vi "digital_bandstop.vi"() -> ()   [LabVIEW 2023]
uses:
  <vilib>/addons/Biomedical/Biosignal Measurements/EEG/EEG FFT Spectrum (Waveform).vi
  <vilib>/addons/Biomedical/NI_BMTK_Measurements.lvlib
panel:
  out "EEG FFT Spectrum before filtering":cluster{"f0":dbl, "df":dbl, "S(f)":dbl[]}(graph)
  out "After High-pass: fc = 1 Hz":dynamicdata(graph)
  out "EEG Signal":dynamicdata(graph)
  out "Gamma Wave FFT Spectrum":cluster{"f0":dbl, "df":dbl, "S(f)":dbl[]}(graph)
  out "Beta Wave FFT Spectrum":cluster{"f0":dbl, "df":dbl, "S(f)":dbl[]}(graph)
  out "Alpha Wave FFT Spectrum":cluster{"f0":dbl, "df":dbl, "S(f)":dbl[]}(graph)
  out "Theta Wave FFT Spectrum":cluster{"f0":dbl, "df":dbl, "S(f)":dbl[]}(graph)
  out "Delta Wave FFT Spectrum":cluster{"f0":dbl, "df":dbl, "S(f)":dbl[]}(graph)
  out "FFT Spectrum":cluster{"f0":dbl, "df":dbl, "S(f)":dbl[]}(graph)
  out "Delta Wave":dynamicdata(graph)
  out "Gamma Wave":dynamicdata(graph)
  out "Beta Wave":dynamicdata(graph)
  out "Alpha Wave":dynamicdata(graph)
  out "Theta Wave":dynamicdata(graph)
  out "After Band-stop: fc = 50 Hz":dynamicdata(graph)
  out "After Low-pass: fc = 31 Hz":dynamicdata(graph)
  in  "stop":bool
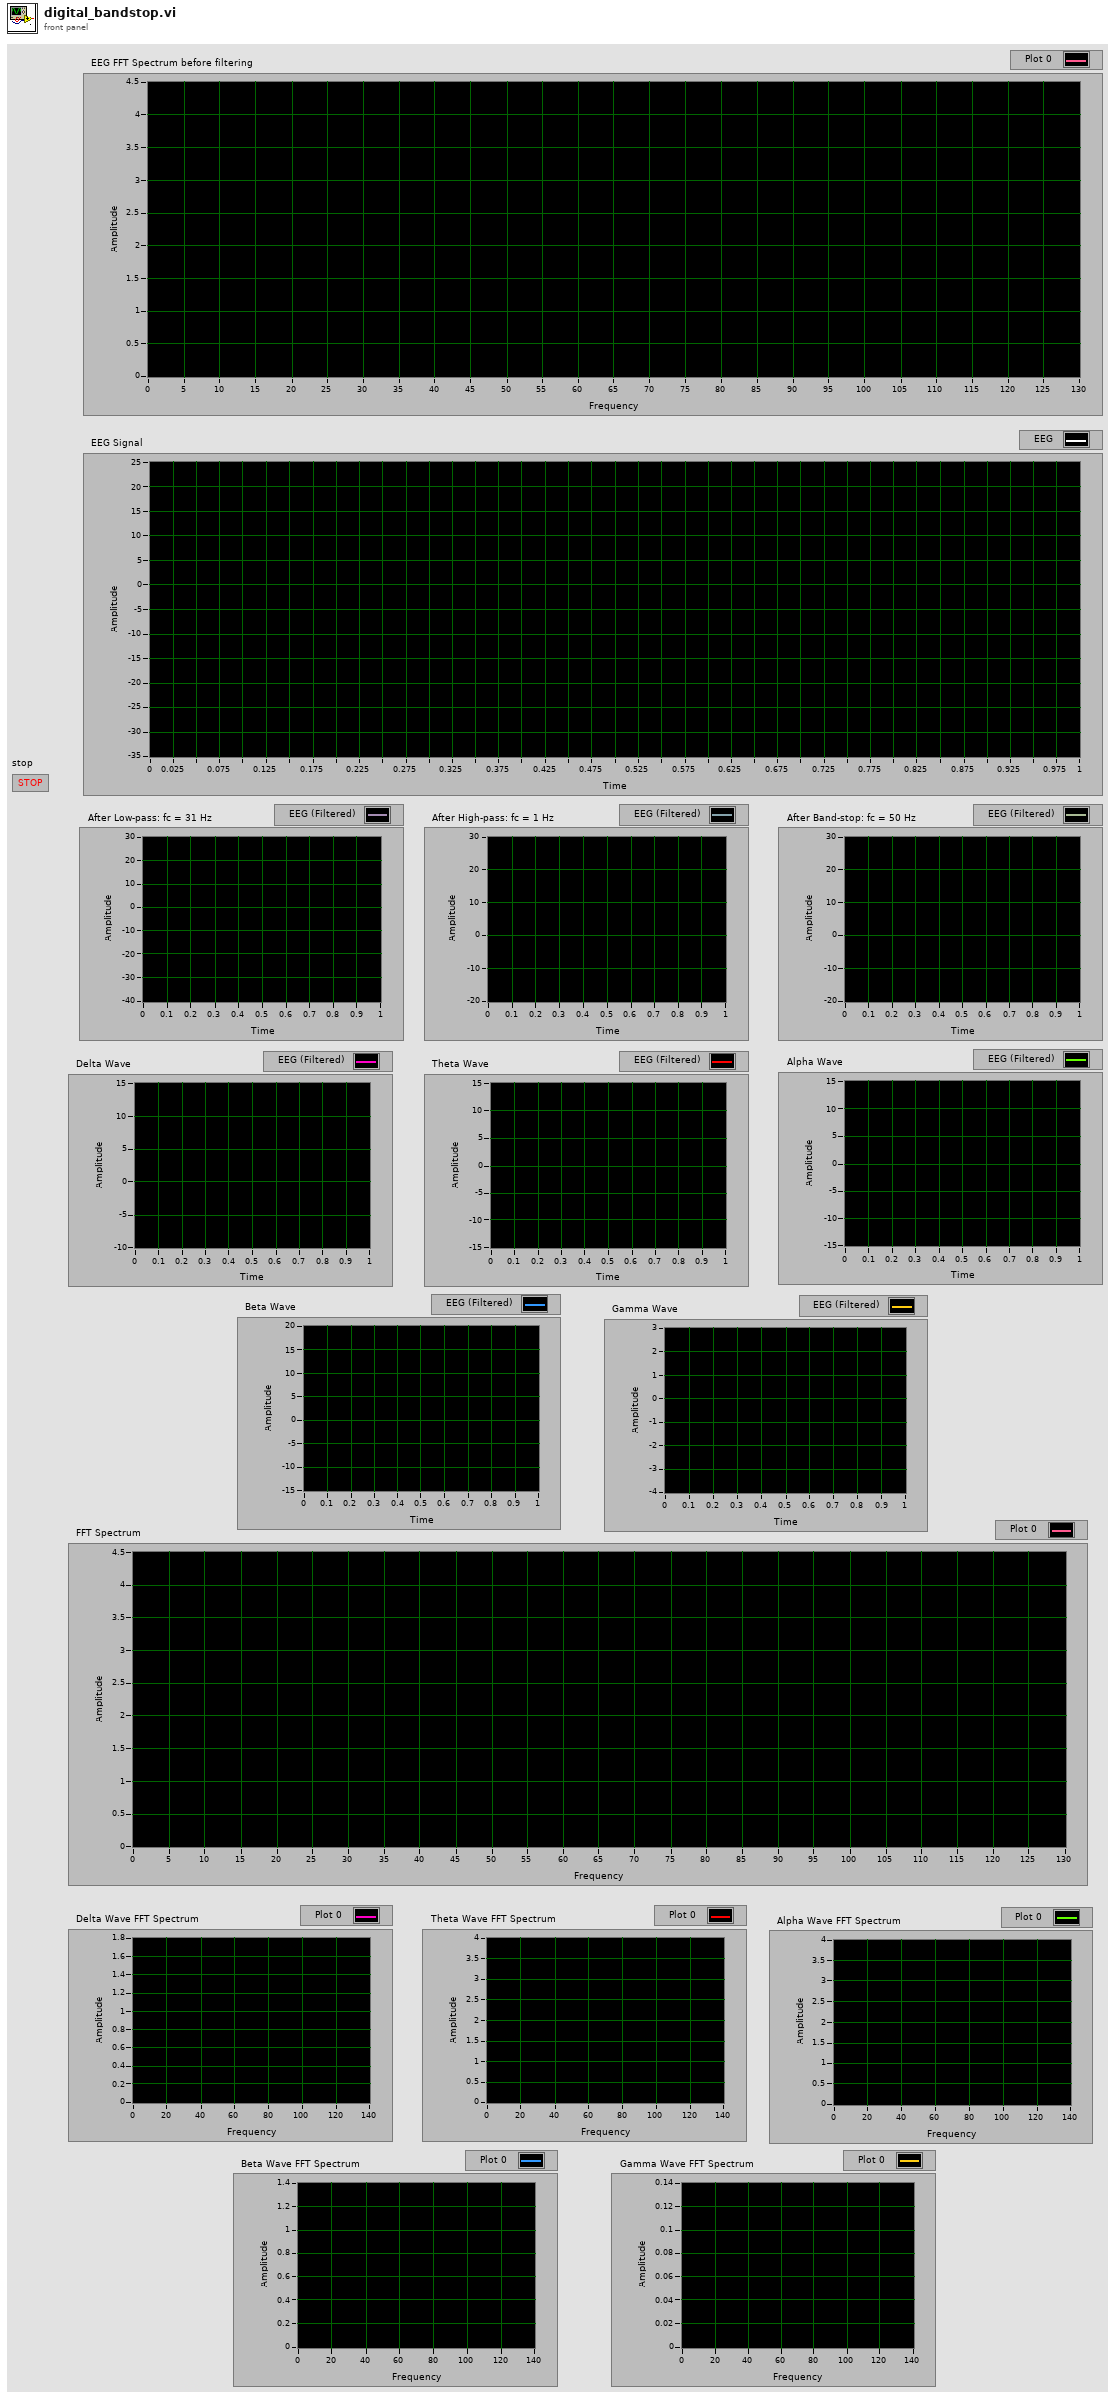
[diagram p1: front panel]
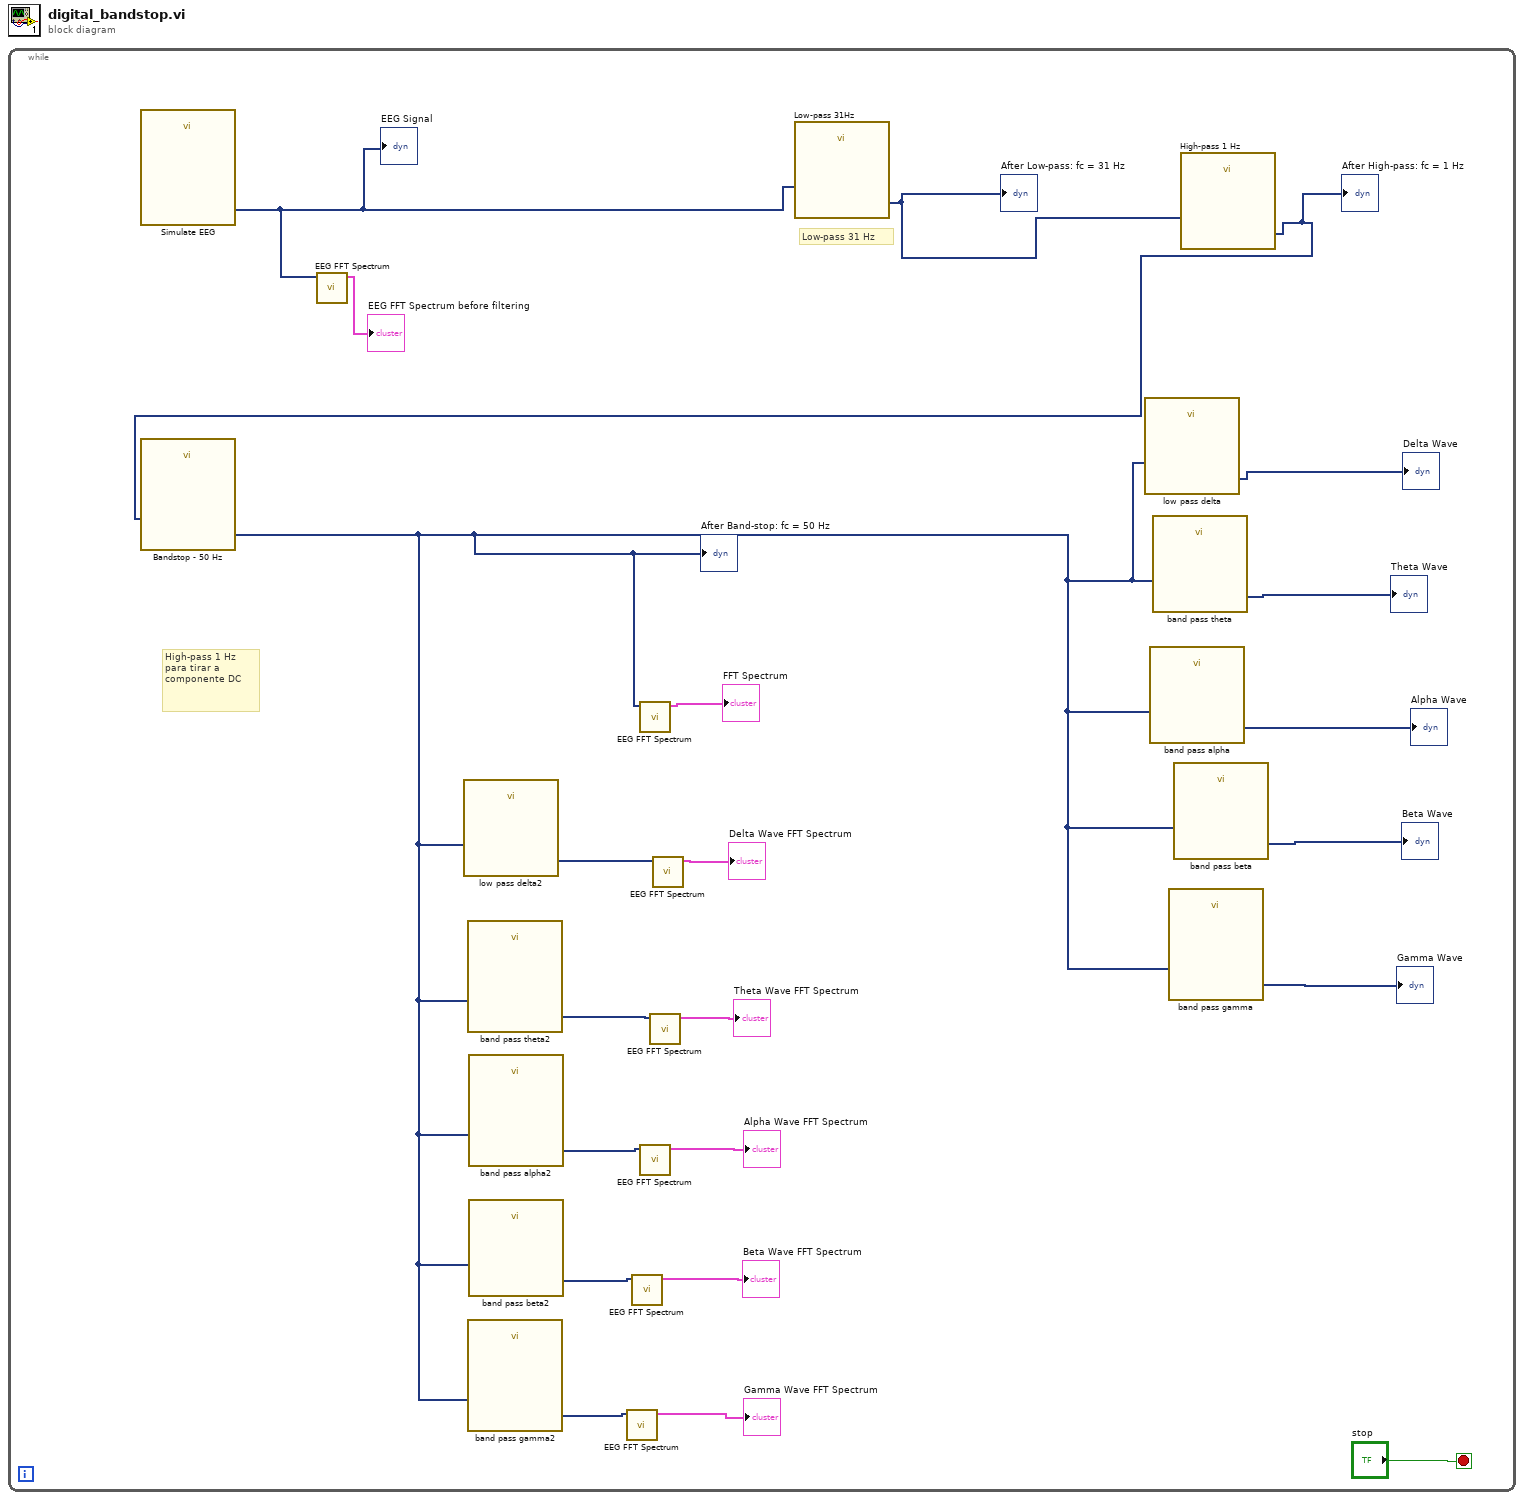
[diagram p0: block diagram]
diagram:
  n1 = while {
    stop <- "stop" stop-if-true
    # "High-pass 1 Hz para tirar a componente DC"
    # "Low-pass 31 Hz"
    n2 = call "Simulate EEG"() -> ("EEG"=w1:dynamicdata)  [unwired: 10 in, 1 out]
    "EEG Signal" <- w1
    n3 = call-poly <vilib>:"EEG FFT Spectrum.vi"("EEG"=w1) -> ("FFT spectrum"=→"EEG FFT Spectrum before filtering":cluster{"f0":dbl, "df":dbl, "S(f)":dbl[]})  [unwired: 8 in, 2 out]
    n4 = call "Low-pass 31Hz"("Signal"=w1) -> ("Filtered Signal"=w21:dynamicdata)  [unwired: 9 in, 1 out]
    "After Low-pass: fc = 31 Hz" <- w21
    n5 = call "High-pass 1 Hz"("Signal"=w21) -> ("Filtered Signal"=w3:dynamicdata)  [unwired: 9 in, 1 out]
    "After High-pass: fc = 1 Hz" <- w3
    n6 = call "Bandstop - 50 Hz"("Signal"=w3) -> ("Filtered Signal"=w4:dynamicdata)  [unwired: 9 in, 1 out]
    "After Band-stop: fc = 50 Hz" <- w4
    n7 = call "low pass delta2"("Signal"=w4) -> ("Filtered Signal"=w13:dynamicdata)  [unwired: 9 in, 1 out]
    n8 = call "band pass theta2"("Signal"=w4) -> ("Filtered Signal"=w12:dynamicdata)  [unwired: 9 in, 1 out]
    n9 = call "band pass gamma2"("Signal"=w4) -> ("Filtered Signal"=w5:dynamicdata)  [unwired: 9 in, 1 out]
    n10 = call "band pass alpha2"("Signal"=w4) -> ("Filtered Signal"=w9:dynamicdata)  [unwired: 9 in, 1 out]
    n11 = call "band pass beta2"("Signal"=w4) -> ("Filtered Signal"=w7:dynamicdata)  [unwired: 9 in, 1 out]
    n12 = call-poly <vilib>:"EEG FFT Spectrum.vi"("EEG"=w5) -> ("FFT spectrum"=→"Gamma Wave FFT Spectrum":cluster{"f0":dbl, "df":dbl, "S(f)":dbl[]})  [unwired: 8 in, 2 out]
    n13 = call-poly <vilib>:"EEG FFT Spectrum.vi"("EEG"=w7) -> ("FFT spectrum"=→"Beta Wave FFT Spectrum":cluster{"f0":dbl, "df":dbl, "S(f)":dbl[]})  [unwired: 8 in, 2 out]
    n14 = call-poly <vilib>:"EEG FFT Spectrum.vi"("EEG"=w4) -> ("FFT spectrum"=→"FFT Spectrum":cluster{"f0":dbl, "df":dbl, "S(f)":dbl[]})  [unwired: 8 in, 2 out]
    n15 = call-poly <vilib>:"EEG FFT Spectrum.vi"("EEG"=w9) -> ("FFT spectrum"=→"Alpha Wave FFT Spectrum":cluster{"f0":dbl, "df":dbl, "S(f)":dbl[]})  [unwired: 8 in, 2 out]
    n16 = call-poly <vilib>:"EEG FFT Spectrum.vi"("EEG"=w12) -> ("FFT spectrum"=→"Theta Wave FFT Spectrum":cluster{"f0":dbl, "df":dbl, "S(f)":dbl[]})  [unwired: 8 in, 2 out]
    n17 = call-poly <vilib>:"EEG FFT Spectrum.vi"("EEG"=w13) -> ("FFT spectrum"=→"Delta Wave FFT Spectrum":cluster{"f0":dbl, "df":dbl, "S(f)":dbl[]})  [unwired: 8 in, 2 out]
    n18 = call "low pass delta"("Signal"=w4) -> ("Filtered Signal"=→"Delta Wave":dynamicdata)  [unwired: 9 in, 1 out]
    n19 = call "band pass alpha"("Signal"=w4) -> ("Filtered Signal"=→"Alpha Wave":dynamicdata)  [unwired: 9 in, 1 out]
    n20 = call "band pass theta"("Signal"=w4) -> ("Filtered Signal"=→"Theta Wave":dynamicdata)  [unwired: 9 in, 1 out]
    n21 = call "band pass gamma"("Signal"=w4) -> ("Filtered Signal"=→"Gamma Wave":dynamicdata)  [unwired: 9 in, 1 out]
    n22 = call "band pass beta"("Signal"=w4) -> ("Filtered Signal"=→"Beta Wave":dynamicdata)  [unwired: 9 in, 1 out]
  }
